vi "AutoPID.vi"(11 "Array":dbl[](array[numeric]) format="%0.3f") -> (0 "output range":cluster{"output high":dbl, "output low":dbl}={"output high"=100.0, "output low"=-100.0} {"output low" format="%.2f"; "output high" format="%.2f"}, 1 "PID gains":T1={"proportional gain (Kc)"=1.0, "integral time (Ti, min)"=0.01, "derivative time (Td, min)"=0.0} {"derivative time (Td, min)" format="%.3f"; "integral time (Ti, min)" format="%.3f"; "proportional gain (Kc)" format="%.3f"})   [LabVIEW 2013]
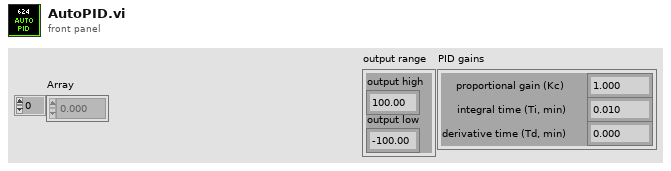
[diagram p1: front panel]
types:
  T1 = cluster{"proportional gain (Kc)":dbl, "integral time (Ti, min)":dbl, "derivative time (Td, min)":dbl}
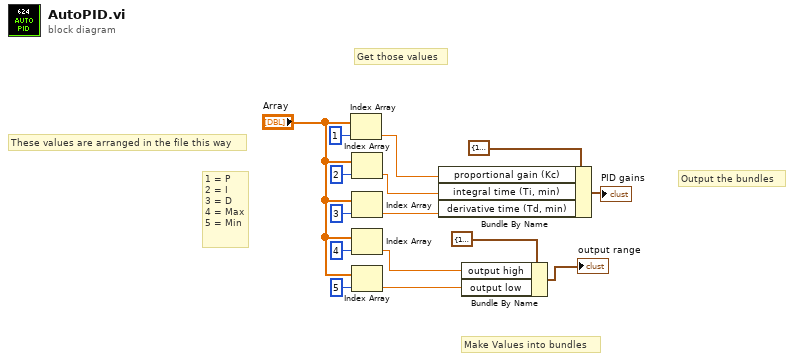
[diagram p0: block diagram]
diagram:
  # "Output the bundles"
  # "Make Values into bundles"
  # "Get those values"
  # "These values are arranged in the file this way"
  # "1 = P\n2 = I\n3 = D\n4 = Max\n5 = Min"
  n1 = Index Array(array="Array", index=1) -> (element=w9:dbl)
  n2 = Index Array(array="Array", index=2) -> (element=w8:dbl)
  n3 = Index Array(array="Array", index=3) -> (element=w7:dbl)
  n4 = Index Array(array="Array", index=4) -> (element=w6:dbl)
  n5 = Index Array(array="Array", index=5) -> (element=w5:dbl)
  n6 = Bundle By Name(cluster=T1 {"proportional gain (Kc)"=1.0, "integral time (Ti, min)"=0.01, "derivative time (Td, min)"=0.0} ("PID gains"), "proportional gain (Kc)"=w9, "integral time (Ti, min)"=w8, "derivative time (Td, min)"=w7) -> (→"PID gains":T1)
  n7 = Bundle By Name(cluster=cluster{"output high":dbl, "output low":dbl} {"output high"=100.0, "output low"=-100.0} ("output range"), "output high"=w6, "output low"=w5) -> (→"output range":cluster{"output high":dbl, "output low":dbl})
